vi "subsystem_salProcessor.vi"(8 "error in (no error)":errorcluster, 10 "topic":string="Start", 11 "ProgrammaticInitialization in":refnum<class "ProgrammaticInitialization.lvclass">) -> (0 "error out":errorcluster, 3 "ProgrammaticInitialization out":refnum<class "ProgrammaticInitialization.lvclass">)   [LabVIEW 2016, in "ProgrammaticInitialization.lvclass"]
uses:
  ProgrammaticInitialization.lvclass
  commandType.ctl
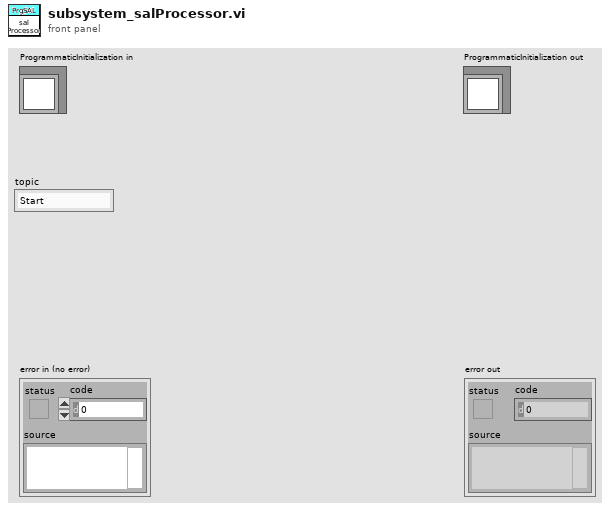
[diagram p1: front panel]
types:
  T1 = typedef "ProgrammaticInitialization.lvclass/commandType.ctl" = enum16{"acceptCommand", "ackCommand", "cancelCallback_command", "cancelCallback_logEvent", "cancelCallback", "flushSamplesEvent", "getEvent", "getNextSample", "getResponse", "getSample", "issueCommand", "logEvent", "monitorCommand", "putSample", "registerCallback_command", "registerCallback_logEvent", "registerCallback", "salCommander", "salEvent", "salProcessor", "salTelemetrySub", "waitForCompletion"}
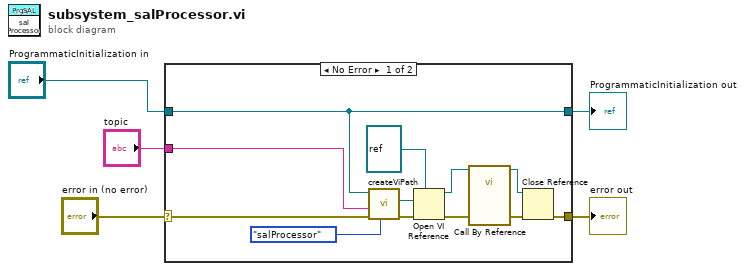
[diagram p0: block diagram]
diagram:
  n1 = case shown="No Error" "error in (no error)" {
    selector: "error in (no error)" -> [w8 w19]
    tunnel: [w7 w19] -> w4
    tunnel: [w9 w18] -> w2
    tunnel: "ProgrammaticInitialization in" -> [w9 w18]
    tunnel: "topic" -> [w10 _]
    frame No Error {
      n2 = call "createViPath.vi"("CommandType"=commandType."salProcessor", "error in (no error)"=w8, "topic"=w10, "ProgrammaticInitialization in"=w9) -> ("error out"=w12:errorcluster, "path"=w11:path)  [unwired: 4 in, 2 out]
      n3 = Open VI Reference(type specifier VI Refnum (for type only)=refnum<vi> refnum, vi path=w11, error in (no error)=w12) -> (vi reference=w13:refnum<vi>, error out=w15:errorcluster)  [unwired: 3 in]
      n4 = call-by-ref "?"(reference=w13, "error in (no error)"=w15) -> (reference out=w14:refnum<vi>, "error out"=w16:errorcluster)  [unwired: 10 in, 2 out]
      n5 = Close Reference(reference=w14, error in (no error)=w16) -> (error out=w7:errorcluster)
    }
    frame Error {
    }
  }
  "error out" <- w4
  "ProgrammaticInitialization out" <- w2
